vi "ModelRead.vi"(8 "error in (no error)":errorcluster, 9 "Save Path":string="C:\\AVC-BarCode\\Save Date\\", 10 "file path (dialog if empty)":path=path "C:/AVC-BarCode/Setting Data/Model.csv", 11 "Data In":T1) -> (0 "error out":errorcluster, 1 "CARNO":u16, 3 "Data Out":T1)   [LabVIEW 2014]
uses:
  controls/Data1.ctl
  controls/Payjson.ctl
  <vilib>/Utility/file.llb/Read From Spreadsheet File (string).vi
panel:
  out "dup path":path
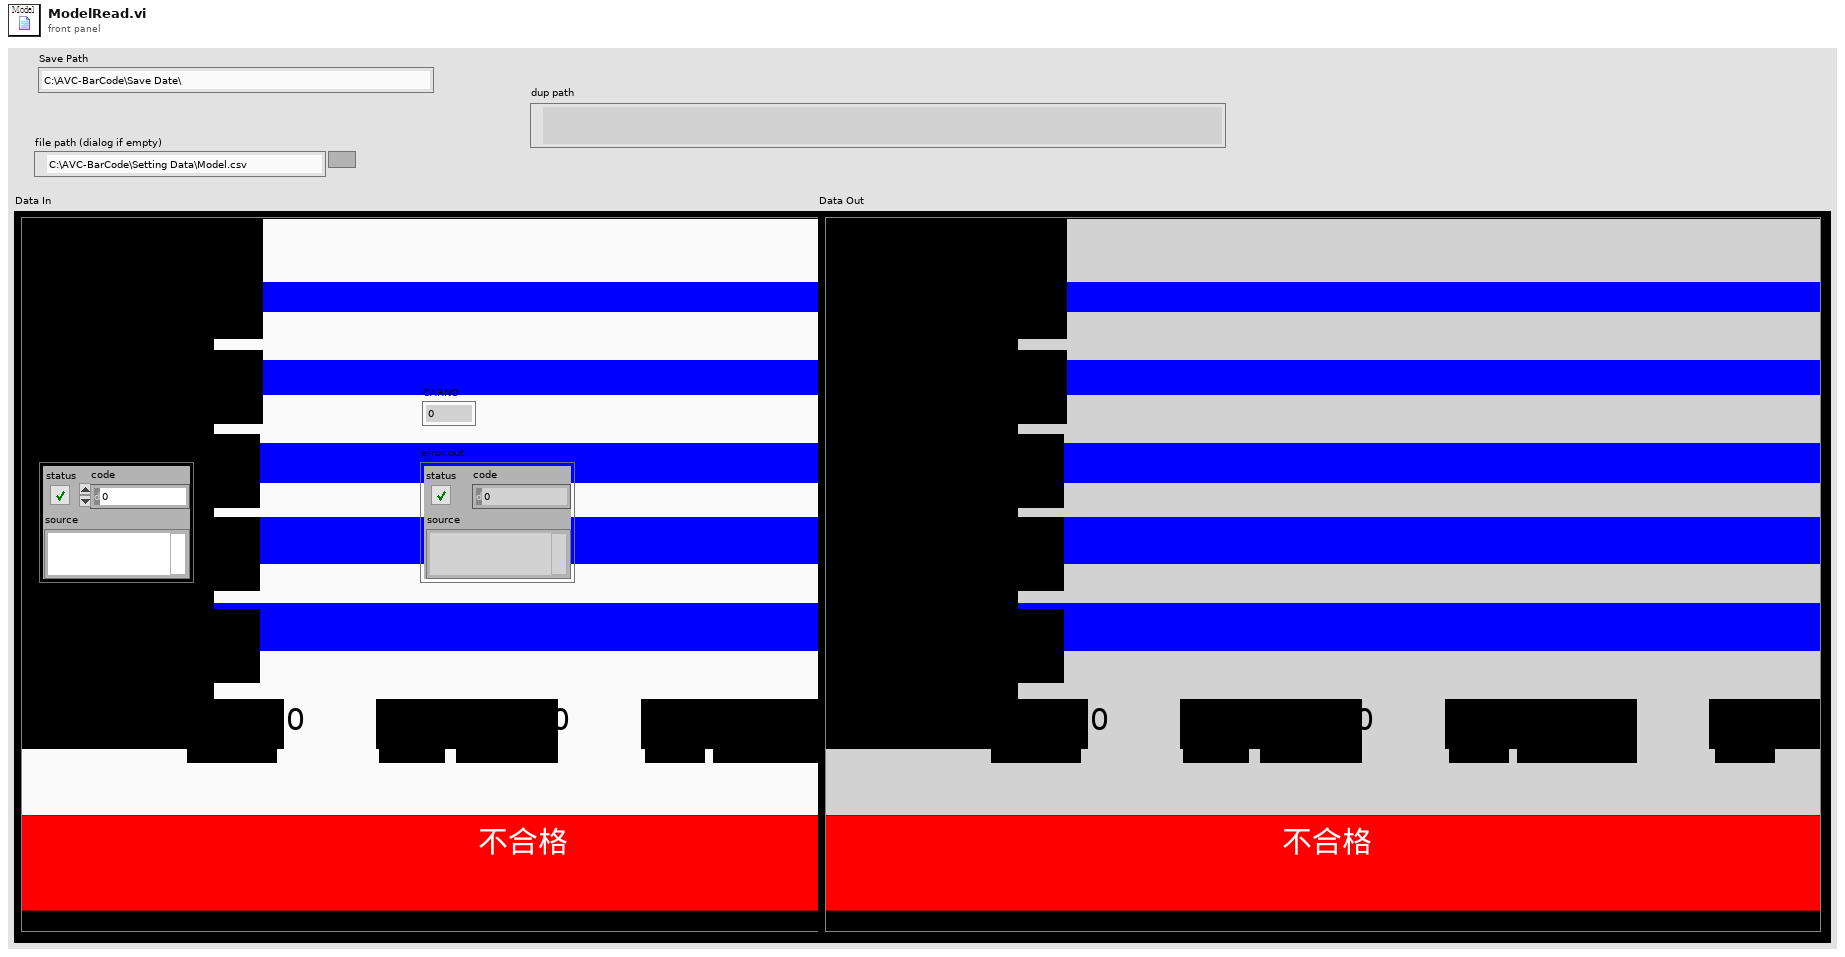
[diagram p1: front panel]
types:
  T1 = typedef "Data1.ctl" = cluster{"Date":string, "BarCode1":string, "BarCode2":string, "BarCode3":string, "Message":string, "OK Count":u16, "NG Count":u16, "Total Count":u16, "ModelData":string[][], "OK&NG":bool, "COM1":refnum<visa-resource-name>, "COM2":refnum<visa-resource-name>, "IO":i32, "Time":u32, "TCP":refnum<k5>, "TCP 2":refnum<k5>, "COM1 2":refnum<visa-resource-name>, "CheckNum":string, "BarCode1_1":string, "BarCode2_1":string, "BarCode3_1":string, "日期":string, "機種":string, "機號":string, "商品條碼1":string, "OK_1":string, "OK":string, "NG":string, "NG_1":string, "Total":string, "Total_1":string, "ClaerTime":u32, "Pjson":T2, "LotNo":string[], "CheckParsArray":string[], "BarCode4":string, "BarCode4_1":string, "商品條碼2":string, "BarCode5":string, "BarCode5_1":string, "商品條碼3":string, "ReScanNG":i32, "NGTimeCT":u32}
  T2 = typedef "Payjson.ctl" = cluster{"DEPT":string, "LINE":string, "STANO":string, "WORKNO":string, "PRODSN":string, "COMPNTID":string, "COMPNTLOT":string, "COMPNTSN":string, "USEDQTY":i16, "OPDATE":string, "OPUSER":string, "RECVDATE":string, "MMODU":string}[]
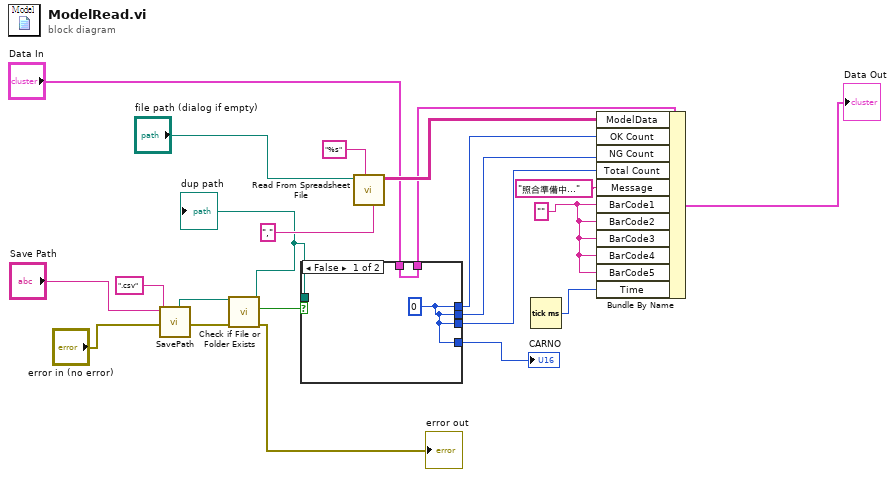
[diagram p0: block diagram]
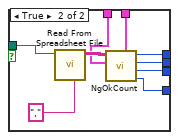
[diagram p2: hidden frame]
diagram:
  w3 = ""
  n1 = call "SavePath.vi"("File Name"=".csv", "Path In"="Save Path") -> ("File Path"=w5:path)  [unwired: 8 in, 1 out]
  n2 = call <vilib>:"Check if File or Folder Exists.vi"("error in (no error)"="error in (no error)", "path"=w5) -> ("error out"=→"error out":errorcluster, "file or folder exists?"=w18:bool, "dup path"=w17:path)  [unwired: 7 in]
  "dup path" <- w17
  n3 = case shown="False" w18 {
    tunnel: w17 -> [_ w32]
    tunnel: [w23 w29] -> w14
    tunnel: [w23 w28] -> w13
    tunnel: [w23 w27] -> w12
    tunnel: [w23 w26] -> w6
    tunnel: "Data In" -> [w22 w25]
    tunnel: [w22 w24] -> w1
    frame False {
      w23 = u16 0 ("OK")
    }
    frame True {
      n4 = call-poly <vilib>:"Read From Spreadsheet File.vi"("delimiter (\\t)"="," ("delimiter (\\t)"), "file path (dialog if empty)"=w32) -> ("all rows"=w30:string[][])  [unwired: 5 in, 4 out]
      n5 = call "NgOkCount.vi"("Data In"=w25, "Data Table In"=w30) -> ("CARNO"=w26:u16, "Total"=w27:u16, "NG"=w28:u16, "OK"=w29:u16, "Data Out"=w24:T1)  [unwired: 5 in]
    }
  }
  "CARNO" <- w6
  n6 = call-poly <vilib>:"Read From Spreadsheet File.vi"("delimiter (\\t)"="," ("delimiter (\\t)"), "format (%s)"="%s", "file path (dialog if empty)"="file path (dialog if empty)") -> ("all rows"=w15:string[][])  [unwired: 4 in, 4 out]
  n7 = Tick Count (ms)() -> (millisecond timer value=w4:u32)
  n8 = Bundle By Name(cluster=w1, "ModelData"=w15, "OK Count"=w14, "NG Count"=w13, "Total Count"=w12, "Message"="照合準備中...", "BarCode1"=w3, "BarCode2"=w3, "BarCode3"=w3, "BarCode4"=w3, "BarCode5"=w3, "Time"=w4) -> (→"Data Out":T1)
